vi "主程序.vi"() -> ()   [LabVIEW 2016]
panel:
  out "波形图":dbl[](graph)
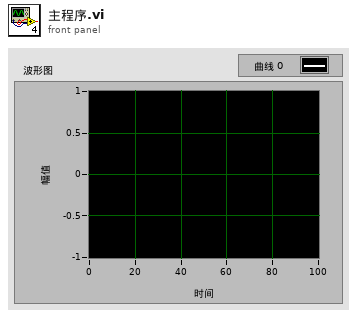
[diagram p1: front panel]
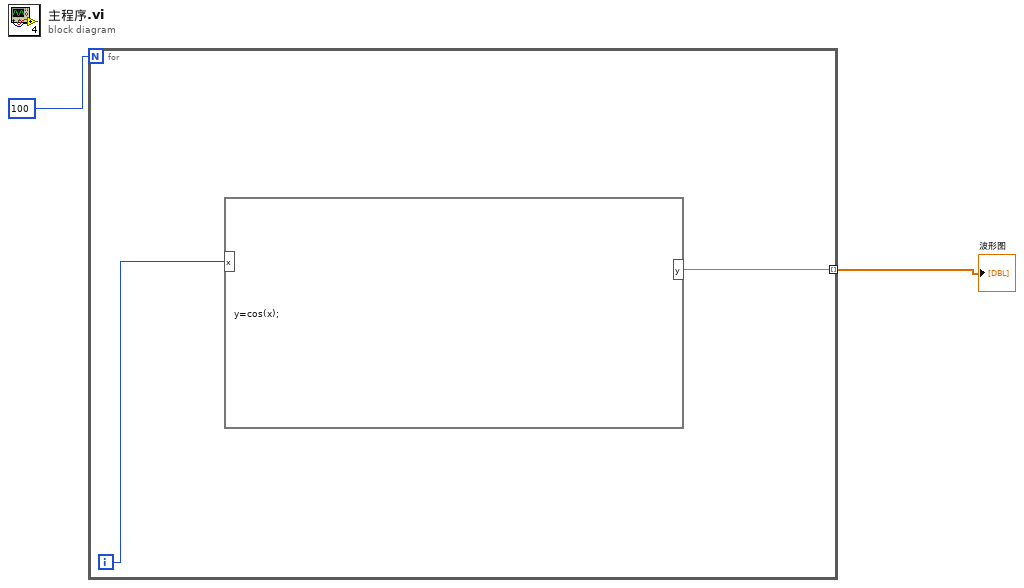
[diagram p0: block diagram]
diagram:
  n1 = for {
    N: 100 -> [_]
    tunnel: [w3] -> w1 mode=indexing
    i -> [w4]
    n2 = formula code="y=cos(x);"("x"=w4) -> ("y"=w3:dbl)
  }
  "波形图" <- w1
